vi "Acquire.vi"(8 "error in (no error)":cluster{"状态":bool, "代码":i32, "源":string} caption="错误输入（无错误）", 9 "数据队列":refnum<queue>, 10 "数据通知器":refnum<notifier>, 11 "硬件资源输入":T1) -> (0 "error out":cluster{"状态":bool, "代码":i32, "源":string} caption="错误输出", 3 "硬件资源输出":T1)   [LabVIEW 2013, in "Acquisition.lvlib"]
doc: "执行采集。替换程序框图的内容，添加对采集硬件的调用。"
uses:
  Acquisition.lvlib
  Hardware Configuration.ctl
  Signal Type.ctl
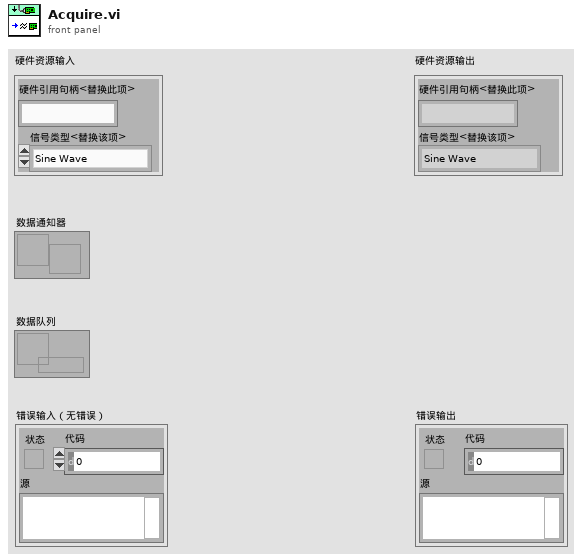
[diagram p1: front panel]
types:
  T1 = typedef "Acquisition.lvlib/Hardware Configuration.ctl" = cluster{"硬件引用句柄<替换此项>":string, "信号类型<替换该项>":T2}
  T2 = typedef "Acquisition.lvlib/Signal Type.ctl" = enum16{"Sine Wave", "Square with Noise"}
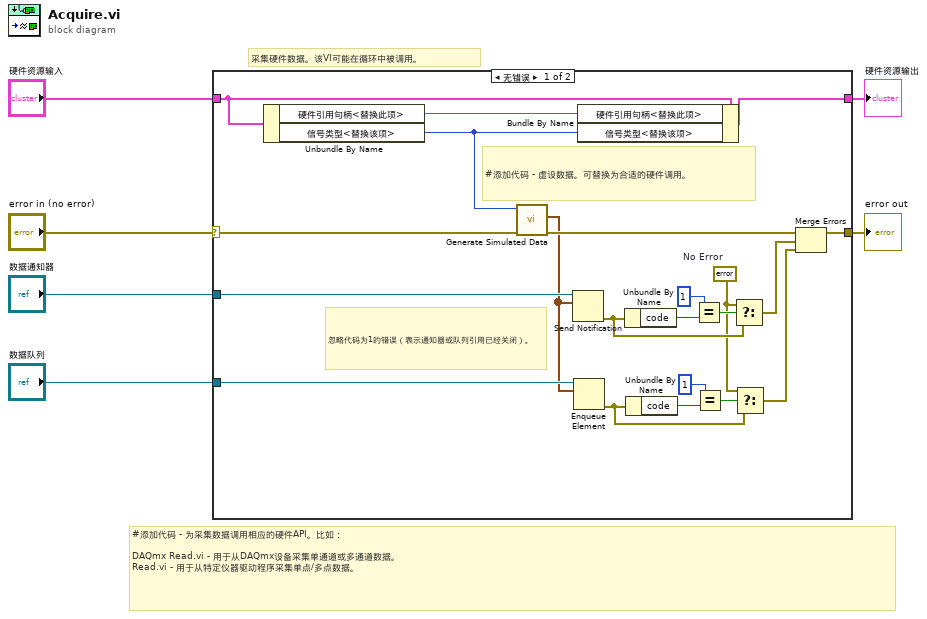
[diagram p0: block diagram]
diagram:
  # "采集硬件数据。该VI可能在循环中被调用。"
  # "#添加代码 - 为采集数据调用相应的硬件API。比如：\n\nDAQmx Read.vi - 用于从DAQmx设备采集单通道或多通道数据。\nRead.vi - 用于从特定仪器驱动程序采集单点/多点数据。"
  n1 = case shown="无错误" "error in (no error)" {
    selector: "error in (no error)" -> [w25 w28]
    tunnel: [w26 w28] -> w5
    tunnel: "硬件资源输入" -> [w21 w29]
    tunnel: [w27 w29] -> w3
    tunnel: "数据通知器" -> [w20 _]
    tunnel: "数据队列" -> [w9 _]
    frame No Error {
      w7 = errorcluster {"status"=FALSE, "code"=0, "source"=""}  # No Error
      # "忽略代码为1的错误（表示通知器或队列引用已经关闭）。"
      # "#添加代码 - 虚设数据。可替换为合适的硬件调用。"
      n2 = Unbundle By Name(w21) -> ("硬件引用句柄<替换此项>"=w22:string, "信号类型<替换该项>"=w23:T2)
      n3 = call "Generate Simulated Data.vi"("error in (no error)"=w25, "信号类型"=w23) -> ("error out"=w24:cluster{"状态":bool, "代码":i32, "源":string}, "图形数据"=w8:waveform(dbl)[])  [unwired: 8 in]
      n4 = Send Notification(notification=w8, notifier=w20) -> (error out=w16:errorcluster)  [unwired: 1 in, 1 out]
      n5 = Enqueue Element(queue=w9, element=w8) -> (error out=w14:errorcluster)  [unwired: 2 in, 2 out]
      n6 = Bundle By Name(cluster=w21, "硬件引用句柄<替换此项>"=w22, "信号类型<替换该项>"=w23) -> (w27:T1)
      n7 = Unbundle By Name(w16) -> ("code"=w19:i32)
      n8 = Unbundle By Name(w14) -> ("code"=w11:i32)
      n9 = Equal?(x=1, y=w19) -> (x = y?=w17:bool)
      n10 = Equal?(x=1, y=w11) -> (x = y?=w13:bool)
      n11 = Select(t=w7, s=w17, f=w16) -> (s? t:f=w15:errorcluster)
      n12 = Select(t=w7, s=w13, f=w14) -> (s? t:f=w10:errorcluster)
      n13 = Merge Errors(w24, w15, w10) -> (w26:errorcluster)
    }
    frame Error {
    }
  }
  "硬件资源输出" <- w3
  "error out" <- w5
